vi "Digital Pin Mode Control.vi"() -> ()   [LabVIEW 2011, in "LVH-LINX.lvlib"]
uses:
  LVH-LINX.lvlib
  Private/Device/Type Defs/Digital Pin Mode.ctl
panel:
  in  "Digital Pin Mode":cluster{"Pin Number":u8, "Digital Pin Mode":T1}
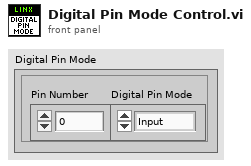
[diagram p1: front panel]
types:
  T1 = typedef "LVH-LINX.lvlib/Digital Pin Mode.ctl" = enum8{"Input", "Output"}
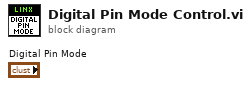
[diagram p0: block diagram]
diagram:
